vi "Write Poll Interval (ms).vi"(8 "error in (no error)":errorcluster, 10 "Poll Interval (ms)":i32=10, 11 "Polled_EventSource in":refnum<class "Polled_EventSource.lvclass">) -> (0 "error out":errorcluster, 3 "Polled_EventSource out":refnum<class "Polled_EventSource.lvclass">)   [LabVIEW 2021, in "Polled_EventSource.lvclass"]
uses:
  Polled_EventSource.lvclass
  Polled_EventSource.lvclass/Polled_EventSource.ctl
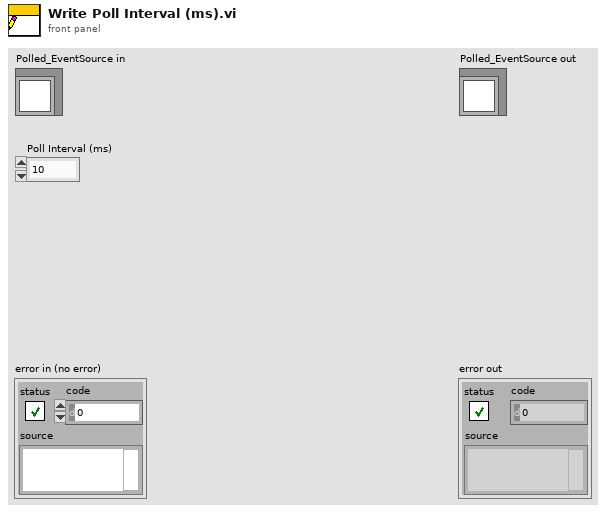
[diagram p1: front panel]
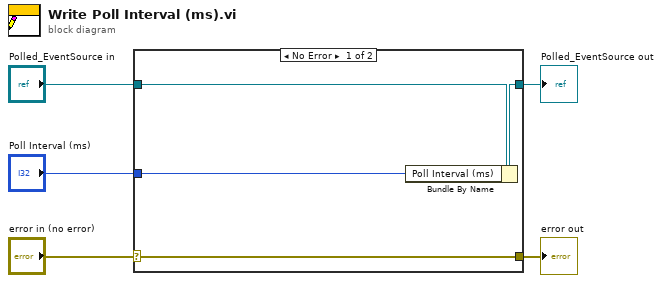
[diagram p0: block diagram]
diagram:
  n1 = case shown="No Error" "error in (no error)" {
    selector: "error in (no error)" -> [w9 w10]
    tunnel: [w9 w10] -> w4
    tunnel: [w7 w11] -> w2
    tunnel: "Polled_EventSource in" -> [w8 w11]
    tunnel: "Poll Interval (ms)" -> [w6 _]
    frame No Error {
      n2 = Bundle By Name(cluster=w8, "Poll Interval (ms)"=w6) -> (w7:refnum<class "Polled_EventSource.lvclass">)
    }
    frame Error {
    }
  }
  "error out" <- w4
  "Polled_EventSource out" <- w2
